vi "GT_GpiSns.vi"(1 "Sense":u16, 2 "rtn_In":cluster{"rtn":i16, "Func":string}) -> (0 "rtn_Out":cluster{"rtn":i16, "Func":string})   [LabVIEW 2014]
uses:
  VC6/gts.dll
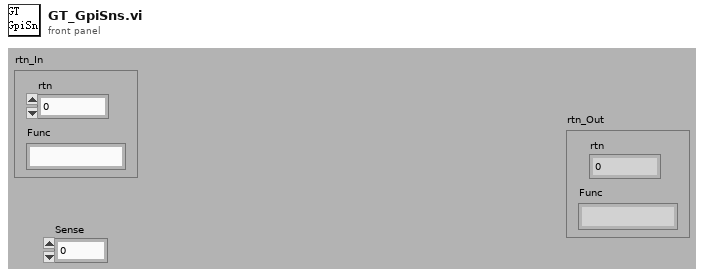
[diagram p1: front panel]
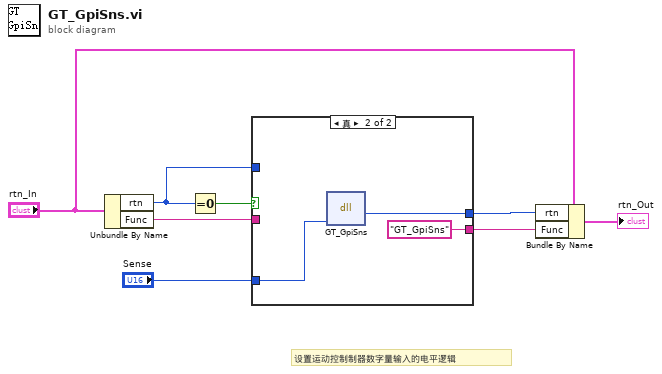
[diagram p0: block diagram]
diagram:
  # "设置运动控制制器数字量输入的电平逻辑"
  n1 = Unbundle By Name("rtn_In") -> ("rtn"=w2:i16, "Func"=w1:string)
  n2 = Equal To 0?(x=w2) -> (x = 0?=w8:bool)
  n3 = case shown="真" w8 {
    tunnel: [w10 w13] -> w5
    tunnel: [w9 "GT_GpiSns" ("Func")] -> w4
    tunnel: "Sense" -> [_ w11]
    tunnel: w2 -> [w10 _]
    tunnel: w1 -> [w9 _]
    frame False {
    }
    frame True {
      n4 = dll-call lib="PTH2Fabs DNewGTS AC-800LWin7版源程序-20170926gts85VC6gts.dll" fn="GT_GpiSns"("Sense"=w11) -> ("rtn"=w13:i16)  [unwired: 4 in, 2 out]
    }
  }
  n5 = Bundle By Name(cluster="rtn_In", "rtn"=w5, "Func"=w4) -> (→"rtn_Out":cluster{"rtn":i16, "Func":string})
